vi "Systematic Error Correction.vi"() -> ()   [LabVIEW 2013]
panel:
  in  "Choose voltmeter":enum16{"V-SIM3", "V-SIM2", "V-SIM1"}(ring)
  out "Результат измерений, В":string
  out "Поправка, В":dbl
  in  "Знаков после зпт":dbl=3.0
  in  "Отн.погр.Rвн %":dbl(slide) min=0.0 max=5.0 step=0.25 scale=0.0..5.0
  out "Показания вольтметра, В":dbl
  in  "Сопротивление источника, Ом":dbl
  in  "Напряжение ИП":T1(ring)
  out "Шкала вольтметра, В":dbl(knob) scale=0.0..4.0
  in  "Выбор предела\nV-SIM1":i32(knob)=8 min=0 max=8 step=1 scale=0.0..8.0
  # "Вычисление и исключение систематической погрешности"
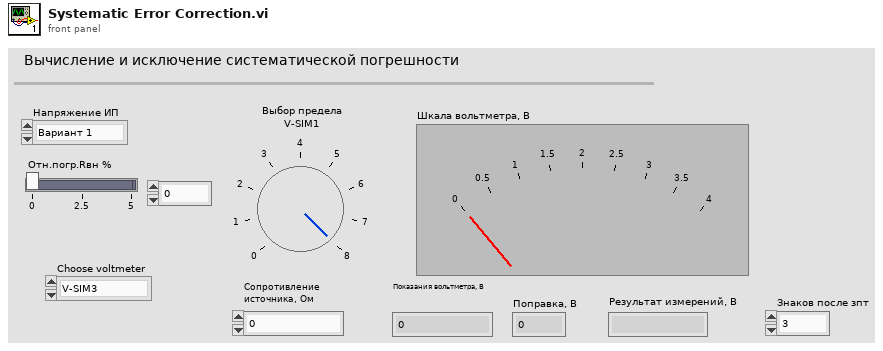
[diagram p1: front panel]
types:
  T1 = enum16{"Вариант 1", "Вариант 2", "Вариант 3", "Вариант 4", "Вариант 5", "Вариант 6", "Вариант 7", "Вариант 8", "Вариант 9", "Вариант 10", "Вариант 11", "Вариант 12"}
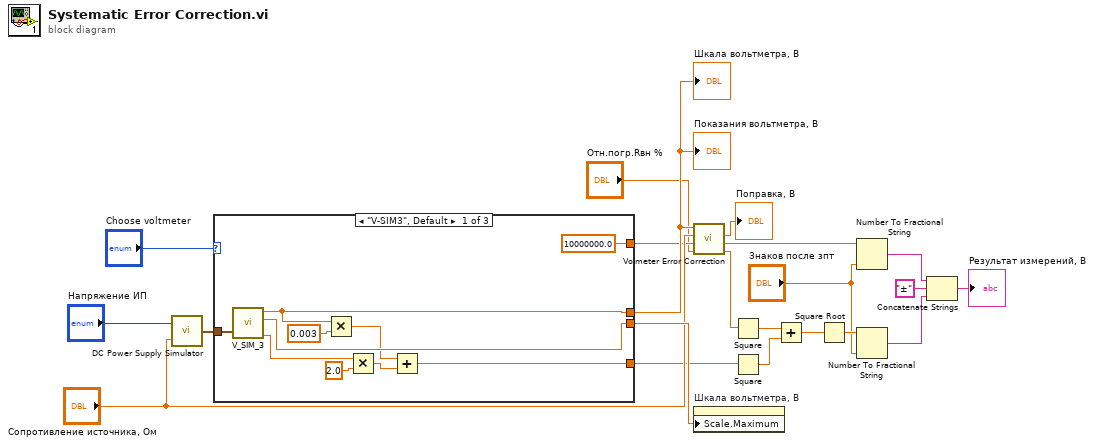
[diagram p0: block diagram]
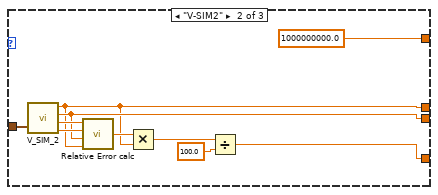
[diagram p2: hidden frame]
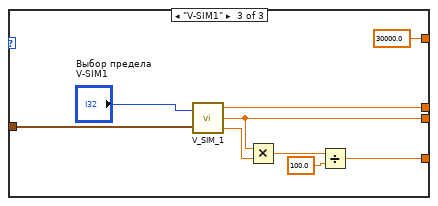
[diagram p3: hidden frame]
diagram:
  n1 = call "DC Power Supply Simulator.vi"("Rвн, Ом"="Сопротивление источника, Ом", "Напряжение ИП"="Напряжение ИП") -> ("Выход"=w20:cluster{"Uип, В":dbl, "Rвн_д, Ом":dbl})
  n2 = case shown="\"V-SIM3\", Default" "Choose voltmeter" {
    tunnel: w20 -> [w31 w41 w50]
    tunnel: [w28 w36 w48] -> w18
    tunnel: [w29 w38 w47] -> w19
    tunnel: [w22 w33 w43] -> w8
    tunnel: [10000000.0 1000000000.0 30000.0] -> w16
    frame "V-SIM3", Default {
      n3 = call "V_SIM_3.vi"("Input"=w31) -> ("Reading (V)"=w28:dbl, "Range (V)"=w29:dbl, "Resolution (V)"=w26:dbl)  [unwired: 2 in]
      n4 = Multiply(x=w28, y=0.003) -> (x*y=w24:dbl)
      n5 = Multiply(x=w26, y=2.0) -> (x*y=w23:dbl)
      n6 = Add(x=w24, y=w23) -> (x+y=w22:dbl)
    }
    frame "V-SIM2" {
      n7 = call "V_SIM_2.vi"("Вход"=w41) -> ("Показания вольтметра, В"=w36:dbl, "Установленный предел, В"=w38:dbl, "c"=w40:dbl, "d"=w39:dbl)  [unwired: 1 in]
      n8 = call "Relative Error calc.vi"("X"=w36, "Xk"=w38, "d"=w39, "C"=w40) -> ("Относительная погрешность, %"=w37:dbl)
      n9 = Multiply(x=w37, y=w36) -> (x*y=w35:dbl)
      n10 = Divide(x=w35, y=100.0) -> (x/y=w33:dbl)
    }
    frame "V-SIM1" {
      n11 = call "V_SIM_1.vi"("Выбор предела измерений"="Выбор предела\nV-SIM1", "Вход"=w50) -> ("Показания вольтметра, В"=w48:dbl, "Установленный предел, В"=w47:dbl, "Класс точности (привед. погр.), %"=w46:dbl)
      n12 = Multiply(x=w47, y=w46) -> (x*y=w45:dbl)
      n13 = Divide(x=w45, y=100.0) -> (x/y=w43:dbl)
    }
  }
  "Шкала вольтметра, В" <- w18
  "Показания вольтметра, В" <- w18
  n14 = call "Volmeter Error Correction.vi"("Относительная погрешность Rвн, %"="Отн.погр.Rвн %", "Rвх вольтметра, Ом"=w16, "Rвн source, Om"="Сопротивление источника, Ом", "Показания вольтметра, В"=w18) -> ("Неисключенная методическа погрешность, В"=w9:dbl, "Исправленные показания,В"=w2:dbl, "Поправка, В"=→"Поправка, В":dbl)  [unwired: 1 out]
  n15 = property on="Шкала вольтметра, В" class="Knob (strict)"("Scale.Maximum"=w19) -> ()  [unwired: 2 in, 2 out]
  n16 = Square(x=w9) -> (x^2=w7:dbl)
  n17 = Square(x=w8) -> (x^2=w6:dbl)
  n18 = Add(x=w7, y=w6) -> (x+y=w5:dbl)
  n19 = Square Root(x=w5) -> (sqrt(x)=w4:dbl)
  n20 = Number To Fractional String(number=w2, precision (6)="Знаков после зпт") -> (F-format string=w12:string)  [unwired: 2 in]
  n21 = Number To Fractional String(number=w4, precision (6)="Знаков после зпт") -> (F-format string=w10:string)  [unwired: 2 in]
  n22 = Concatenate Strings(w12, "±", w10) -> (→"Результат измерений, В":string)
